vi "RSZVB Set Pulse Generator Type.vi"(7 "Pulse Type (0)":i32(ring) items=["Single Pulse", "Pulse Train", "Constant High", "Constant Low"], 8 "error in (no error)":errorcluster {"code" format="%.0x"}, 9 "Generator (1)":i32=1, 10 "Channel (1)":i32=1, 11 "VISA session":refnum<visa-resource-name>) -> (0 "error out":errorcluster {"code" format="%.0x"}, 3 "dup VISA session":refnum<visa-resource-name>)   [LabVIEW 2011]
doc: "This VI selects the pulse type of the pulse generator signal <gen_no>. \n\nNote(s):\n\n(1) This VI is available only with option R&S ZVA-K27.\n\nRemote-control command(s):\n[SENSe<Ch>:]PULSe:GENerator<gen_no>:TYPE SINGle | TRAin | CHIGh | CLOW"
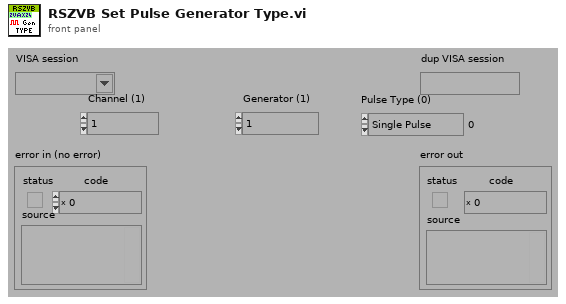
[diagram p1: front panel]
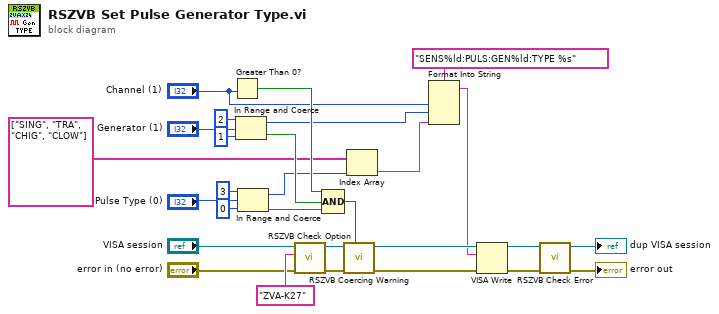
[diagram p0: block diagram]
diagram:
  n1 = Greater Than 0?(x="Channel (1)") -> (x > 0?=w10:bool)
  n2 = In Range and Coerce(upper limit=2, x="Generator (1)", lower limit=1) -> (coerced(x)=w8:i32, In Range?=w11:bool)
  n3 = In Range and Coerce(upper limit=3, x="Pulse Type (0)", lower limit=0) -> (coerced(x)=w7:i32, In Range?=w12:bool)
  n4 = call "RSZVB Check Option.vi"("error in (no error)"="error in (no error)", "Options"="ZVA-K27", "VISA session"="VISA session") -> ("error out"=w22:errorcluster, "dup VISA session"=w21:refnum<visa-resource-name>)  [unwired: 7 in]
  n5 = Compound Arithmetic op=AND(w10, w11, w12) -> (w14:bool)
  n6 = call "RSZVB Coercing Warning.vi"("In Range?"=w14, "error in (no error)"=w22, "VISA session"=w21) -> ("error out"=w27:errorcluster, "dup VISA session"=w28:refnum<visa-resource-name>)  [unwired: 7 in]
  n7 = Index Array(array=string[] ["SING", "TRA", "CHIG", "CLOW"], index=w7) -> (element=w5:string)
  n8 = Format Into String(format string="SENS%ld:PULS:GEN%ld:TYPE %s", "Channel (1)", w8, w5) -> (resulting string=w24:string)  [unwired: 2 in, 1 out]
  n9 = VISA Write(VISA resource name=w28, write buffer=w24, error in (no error)=w27) -> (VISA resource name out=w25:refnum<visa-resource-name>, error out=w26:errorcluster)  [unwired: 1 out]
  n10 = call "RSZVB Check Error.vi"("error in (no error)"=w26, "VISA session"=w25) -> ("error out"=→"error out":errorcluster, "dup VISA session"=→"dup VISA session":refnum<visa-resource-name>)  [unwired: 8 in]
